vi "destroy.vi"(8 "error in (no error)":errorcluster, 11 "Image in":refnum<class "Image.lvclass">) -> (0 "error out":errorcluster, 3 "Image out":refnum<class "Image.lvclass">)   [LabVIEW 2010, in "Image.lvclass"]
uses:
  Image.lvclass
  <vilib>/vision/Image Controls.llb/IMAQ Image.ctl
  ErrorController/ErrorController/class_data.vi
  ErrorController/ErrorController/ErrorController.lvclass
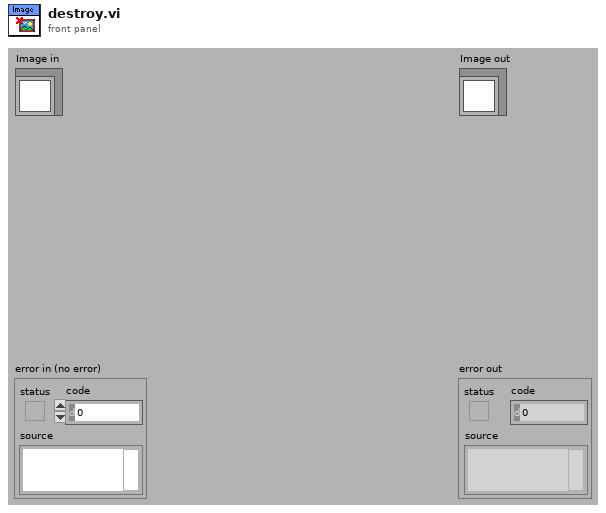
[diagram p1: front panel]
types:
  T1 = typedef "IMAQ Image.ctl" = refnum<image>
  T2 = typedef "Image.lvclass/storage_mode.ctl" = enum16{"RAM", "disk"}
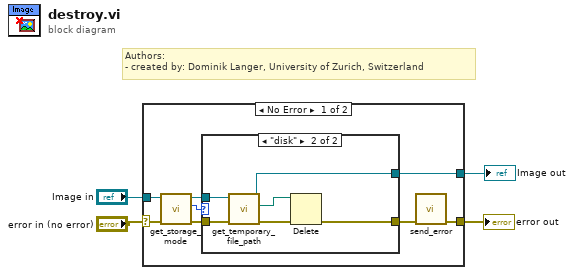
[diagram p0: block diagram]
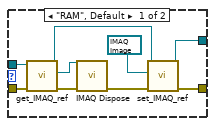
[diagram p2: hidden frame]
diagram:
  # "Authors: \n- created by: Dominik Langer, University of Zurich, Switzerland"
  n1 = case shown="No Error" "error in (no error)" {
    selector: "error in (no error)" -> [w10 w29]
    tunnel: [w6 w29] -> w3
    tunnel: [w7 w28] -> w1
    tunnel: "Image in" -> [w12 w28]
    frame No Error {
      n2 = call-dynamic "get_storage_mode.vi"("error in (no error)"=w10, "Image.lvclass in"=w12) -> ("error out"=w9:errorcluster, "storage mode"=w8:T2, "Image.lvclass out"=w11:refnum<class "Image.lvclass">)  [unwired: 7 out]
      n3 = case shown="\"disk\"" w8 {
        tunnel: [w16 w24] -> w5
        tunnel: w11 -> [w19 w26]
        tunnel: w9 -> [w18 w27]
        tunnel: [w13 w22] -> w7
        frame "RAM", Default {
          n4 = call-dynamic "get_IMAQ_ref.vi"("error in (no error)"=w18, "Image.lvclass in"=w19) -> ("error out"=w21:errorcluster, "Image"=w20:T1, "Image.lvclass out"=w14:refnum<class "Image.lvclass">)  [unwired: 7 out]
          n5 = call "IMAQ Dispose"("Image"=w20, "error in (no error)"=w21) -> ("error out"=w17:errorcluster)  [unwired: 1 in, 3 out]
          n6 = call-dynamic "set_IMAQ_ref.vi"("error in (no error)"=w17, "Image"=T1 refnum ("IMAQ ref"), "Image.lvclass in"=w14) -> ("error out"=w16:errorcluster, "Image.lvclass out"=w13:refnum<class "Image.lvclass">)  [unwired: 7 out]
        }
        frame "disk" {
          n7 = call-dynamic "get_temporary_file_path.vi"("error in (no error)"=w27, "Image.lvclass in"=w26) -> ("error out"=w25:errorcluster, "temporary file path"=w23:path, "Image.lvclass out"=w22:refnum<class "Image.lvclass">)  [unwired: 7 out]
          n8 = Delete(path (use dialog)=w23, error in=w25) -> (error out=w24:errorcluster)  [unwired: 5 out]
        }
      }
      n9 = call "send_error.vi"("error in (no error)"=w5) -> ("error out"=w6:errorcluster)  [unwired: 10 in]
    }
    frame Error {
    }
  }
  "error out" <- w3
  "Image out" <- w1
